vi "BIN-write.vi"(8 "error in":errorcluster, 10 "Data in":T1, 11 "refnum in":refnum<file>) -> (0 "error out":errorcluster)   [LabVIEW 2020, in "DBAL-BIN.lvclass"]
doc: "Write to a Binary historian file"
uses:
  DBAL-BIN.lvclass
  controls/BIN/BINdata.ctl
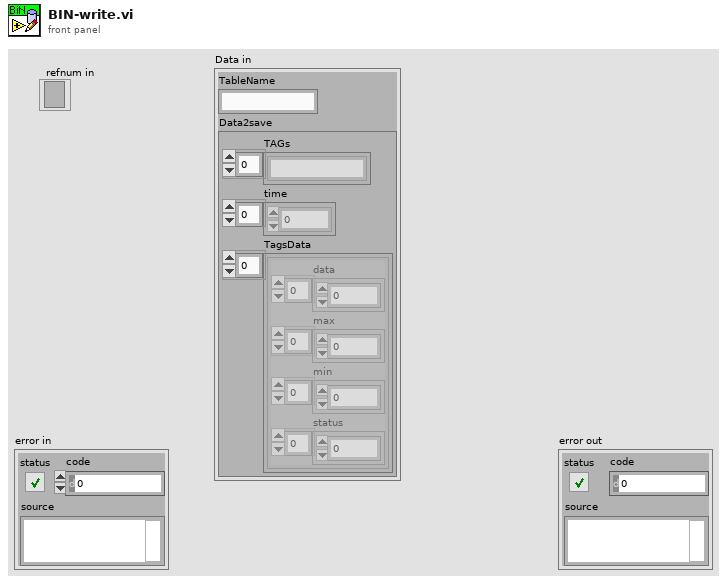
[diagram p1: front panel]
types:
  T1 = cluster{"TableName":string, "Data2save":cluster{"TAGs":string[], "time":dbl[], "TagsData":cluster{"data":dbl[], "max":dbl[], "min":dbl[], "status":u32[]}[]}}
  T2 = enum16{"big-endian, network order", "native, host order", "little-endian"}
  T3 = typedef "DBAL-BIN.lvclass/BINdata.ctl" = cluster{"time":dbl[], "TagsData":cluster{"data":dbl[], "max":dbl[], "min":dbl[], "status":u32[]}[]}
  T4 = cluster{"data":dbl[], "max":dbl[], "min":dbl[], "status":u32[]}[]
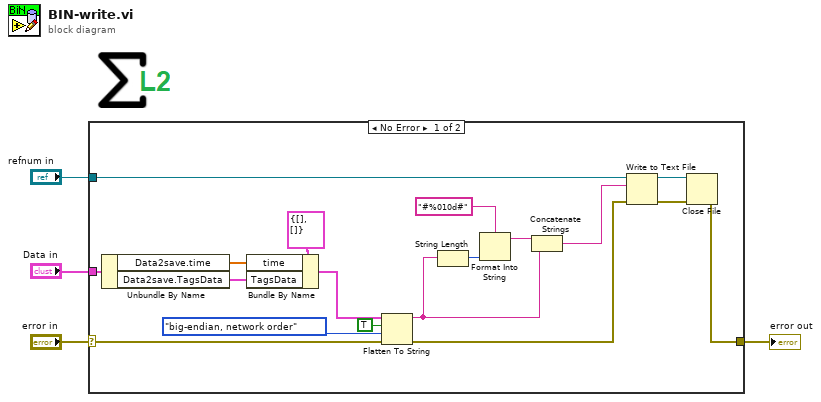
[diagram p0: block diagram]
diagram:
  n1 = case shown="No Error" "error in" {
    selector: "error in" -> [w13 w23]
    tunnel: [w22 w23] -> w3
    tunnel: "refnum in" -> [w8 _]
    tunnel: "Data in" -> [w21 _]
    frame No Error {
      n2 = Unbundle By Name(w21) -> ("Data2save.time"=w19:dbl[], "Data2save.TagsData"=w18:T4)
      n3 = Bundle By Name(cluster=T3 {"time"=[], "TagsData"=[]} ("BinHistData"), "time"=w19, "TagsData"=w18) -> (w6:T3)
      n4 = Flatten To String(anything=w6, prepend array or string size? (T)=TRUE, byte order (0:big-endian, network order)=T2."big-endian, network order", error in (no error)=w13) -> (data string=w5:string, error out=w10:errorcluster)  [unwired: 1 out]
      n5 = String Length(string=w5) -> (length=w17:i32)
      n6 = Format Into String(format string="#%010d#", w17) -> (resulting string=w15:string)  [unwired: 2 in, 1 out]
      n7 = Concatenate Strings(w15, w5) -> (w7:string)
      n8 = Write to Text File(file (use dialog)=w8, text=w7, error in=w10) -> (refnum out=w11:refnum<file>, error out=w12:errorcluster)  [unwired: 1 in, 1 out]
      n9 = Close File(refnum=w11, error in=w12) -> (error out=w22:errorcluster)  [unwired: 1 out]
    }
    frame Error {
    }
  }
  "error out" <- w3
